vi "MAIN.vi"() -> ()   [LabVIEW 2019]
uses:
  TypeDefs/Estados_flujo_Debug.ctl
  TypeDefs/CLUSTER_CONTROLES_INDICADORES.ctl
  TypeDefs/TAREAS.ctl
  SHARED TYPES/Acciones_UI.ctl
  <vilib>/Utility/error.llb/Error Cluster From Error Code.vi
  <vilib>/ErrorRing/Error Ring.xnode
  SHARED TYPES/SHARED TYPES.lvlib
  SHARED VI'S/SHARED VI'S.lvlib
  MOVIMIENTO_CABEZAL/LABVIEW_MOVIMIENTO_ABSOLUTO/MAIN_call.vi
panel:
  in  "Tab Control":enum32{"Page 1", "Page 2"}(tab)
  in  "TEST ASICS":bool
  in  "LEER QR":bool
  out "LABVIEW MESSAGES":string
  in  "MOVER ASICS":bool
  in  "CALIBRACION":bool
  in  "Exit":bool
  in  "INICIAR COM":bool
  out "DISPOSITIVO CONECTADO":string
  out "ARDUINO MESSAGES":string
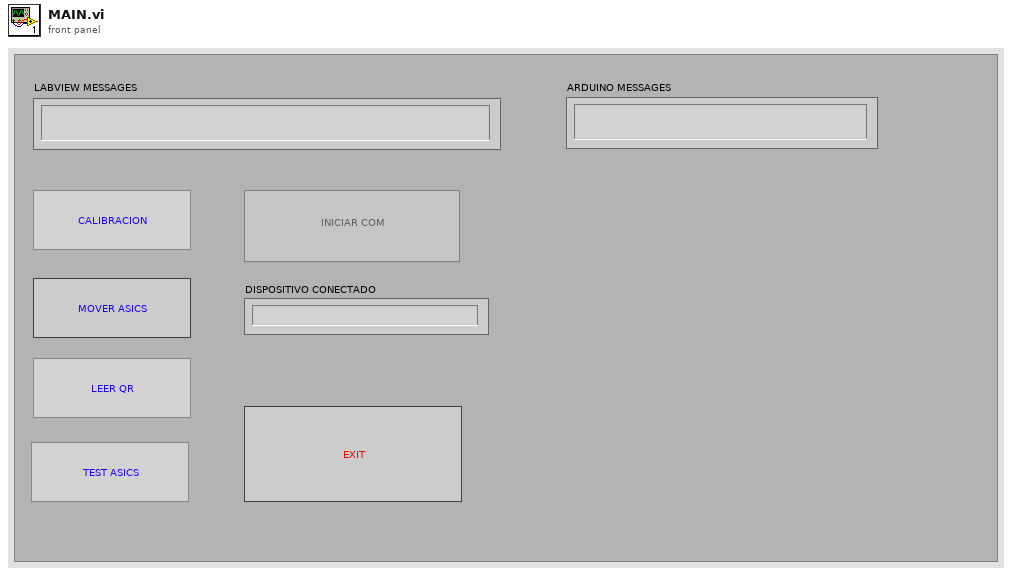
[diagram p1: front panel]
types:
  T1 = typedef "TAREAS.ctl" = enum16{"NINGUNA", "TEST ASICS", "CALIBRACION", "MOVER ASICS", "LEER QR"}
  T2 = typedef "CLUSTER_CONTROLES_INDICADORES.ctl" = cluster{"TEST ASICS":refnum<vi>, "MOVER ASICS":refnum<vi>, "LEER QR'S":refnum<vi>, "MESSAGES":refnum<vi>, "INICIAR COM":refnum<vi>, "stop":refnum<vi>, "CALIBRACION":refnum<vi>}
  T3 = typedef "Estados_flujo_Debug.ctl" = enum16{"Init", "Sesiones Visa abiertas?", "Iniciar Visa Arduino", "Esperar Evento", "Tarea", "Ping to Arduino", "Wait to flag", "Exit", "Error?"}
  T4 = typedef "SHARED TYPES.lvlib/Acciones_UI.ctl" = enum16{"Activar", "Desactivar", "Reiniciar default"}
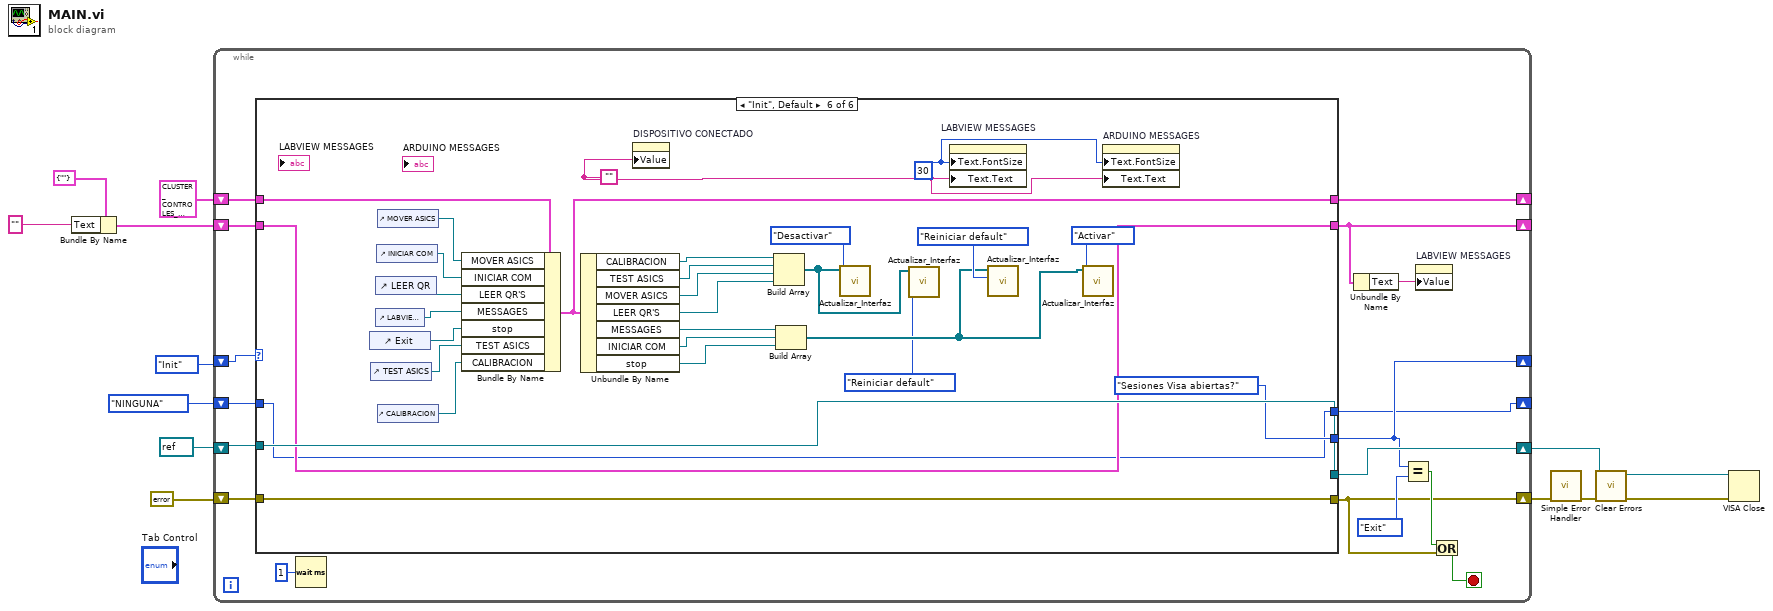
[diagram p0: block diagram]
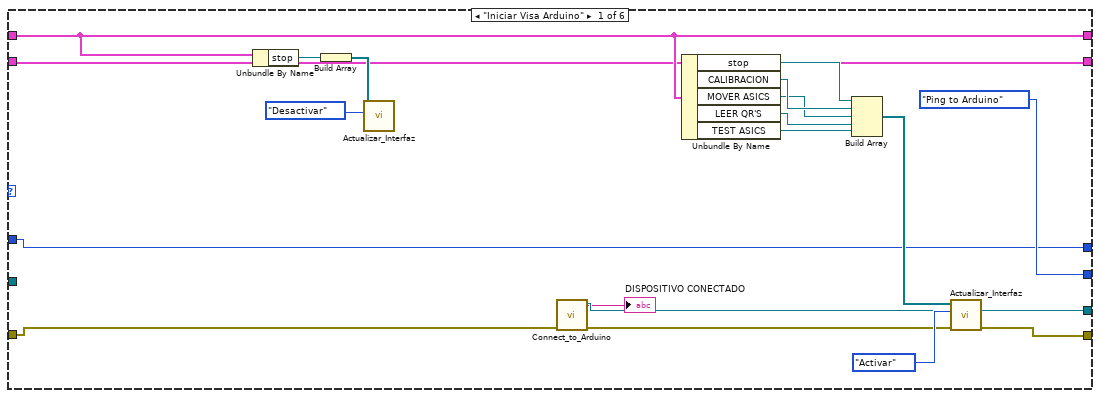
[diagram p2: hidden frame]
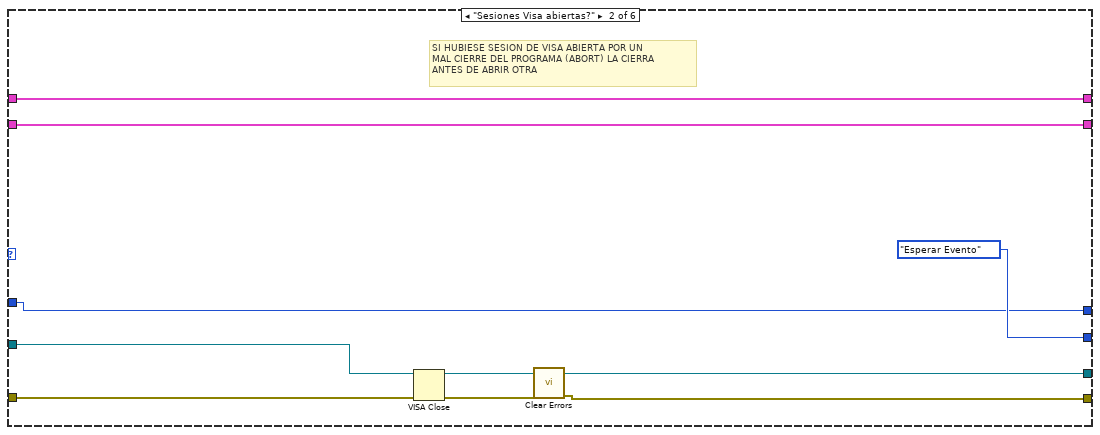
[diagram p3: hidden frame]
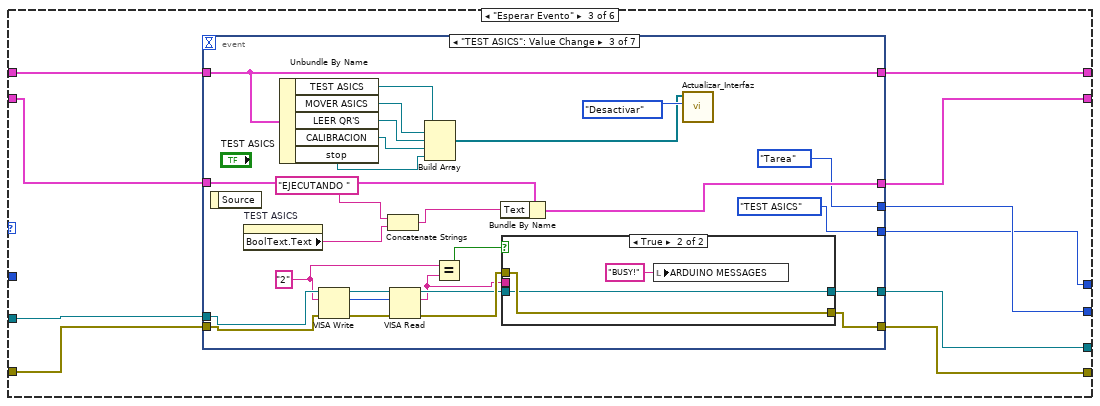
[diagram p4: hidden frame]
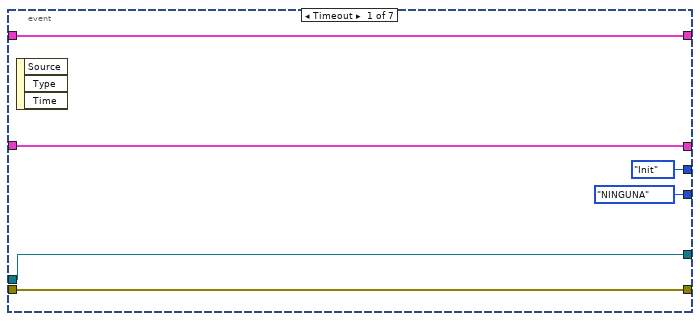
[diagram p5: hidden frame]
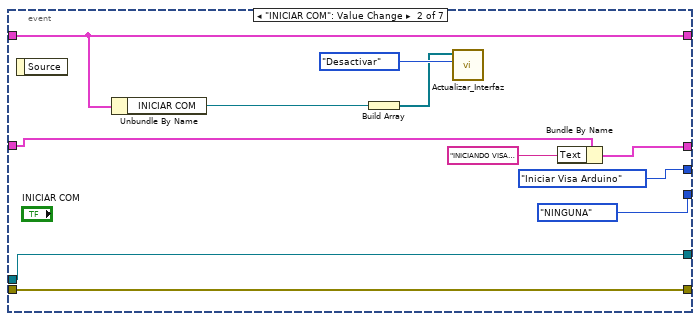
[diagram p6: hidden frame]
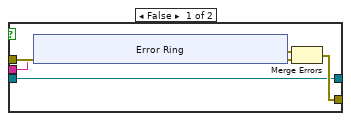
[diagram p7: hidden frame]
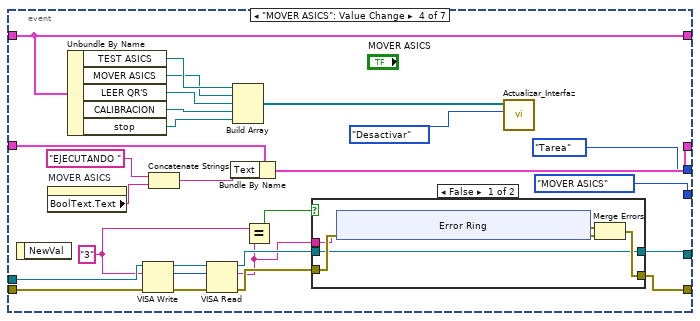
[diagram p8: hidden frame]
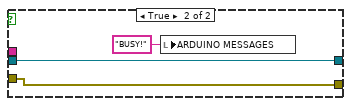
[diagram p9: hidden frame]
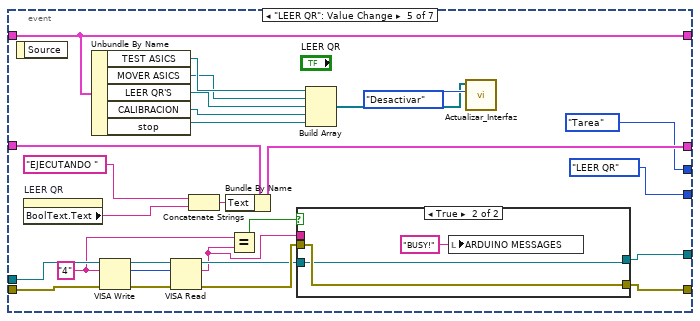
[diagram p10: hidden frame]
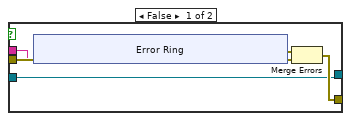
[diagram p11: hidden frame]
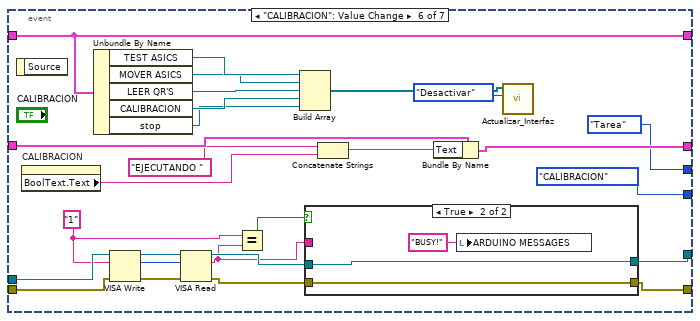
[diagram p12: hidden frame]
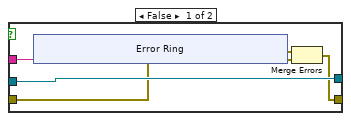
[diagram p13: hidden frame]
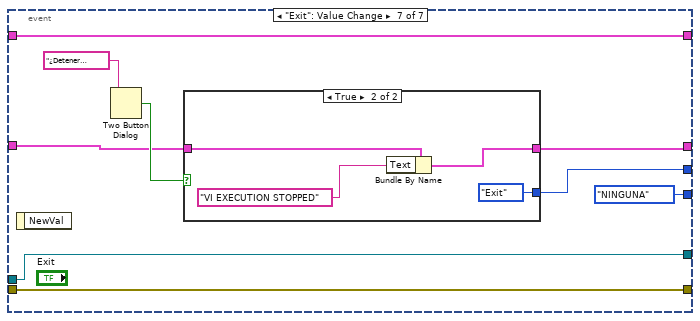
[diagram p14: hidden frame]
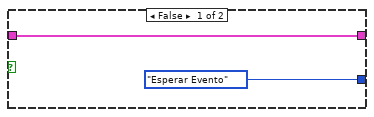
[diagram p15: hidden frame]
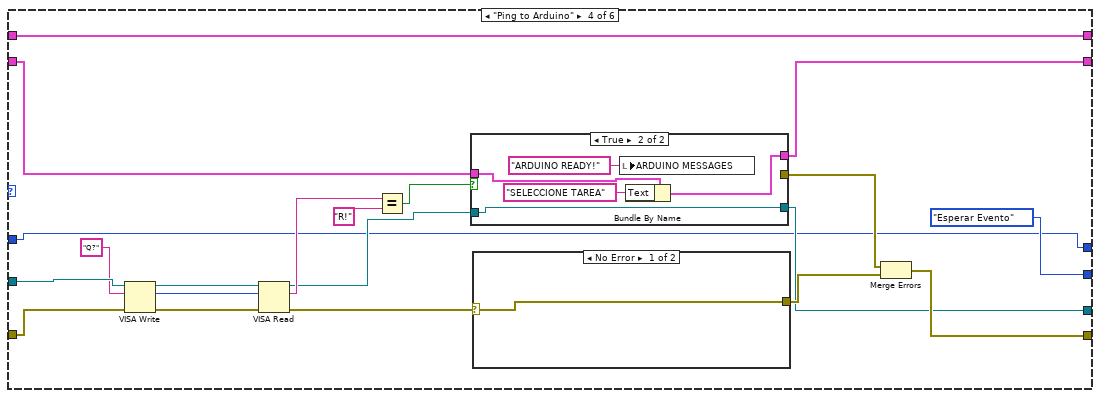
[diagram p16: hidden frame]
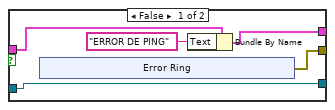
[diagram p17: hidden frame]
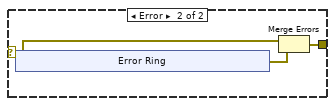
[diagram p18: hidden frame]
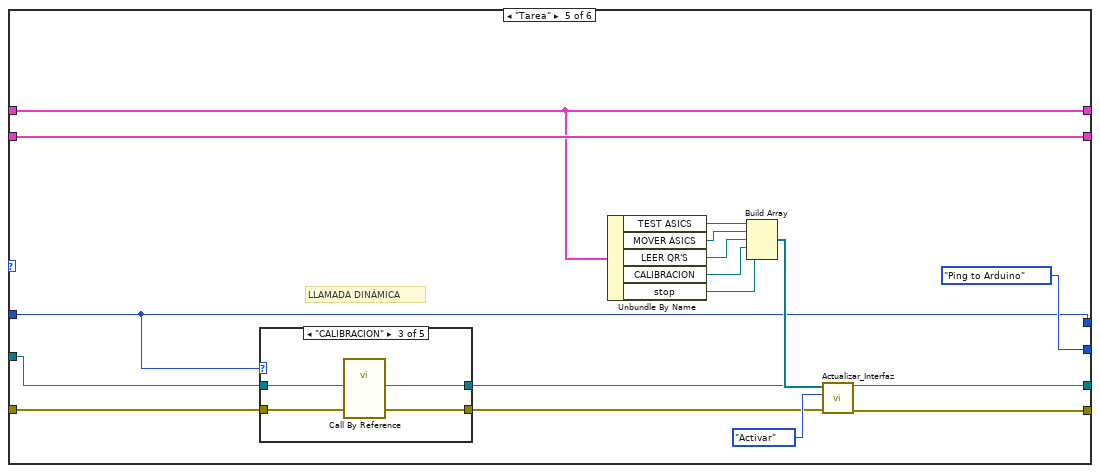
[diagram p19: hidden frame]
diagram:
  n1 = Bundle By Name(cluster=cluster{"Text":string} {"Text"=""}, "Text"="" ("element")) -> (w3:cluster{"Text":string})
  n2 = while {
    shift-right: [w20] -> w7
    shift-left: errorcluster {"status"=FALSE, "code"=0, "source"=""} ("error out") -> [w29]
    shift-right: [w23] -> w11
    shift-left: refnum<visa-resource-name> refnum ("VISA resource name out") -> [w24]
    shift-right: [w25] -> _
    shift-left: T2 {"TEST ASICS"=refnum, "MOVER ASICS"=refnum, "LEER QR'S"=refnum, "MESSAGES"=refnum, "INICIAR COM"=refnum, "stop"=refnum, "CALIBRACION"=refnum} ("INDICADORES_CONTROLES") -> [w26]
    shift-right: [w17] -> _
    shift-left: w3 -> [w19]
    shift-right: [w15] -> _
    shift-left: Estados_flujo_Debug."Init" -> [w16]
    shift-right: [w13] -> _
    shift-left: TAREAS."NINGUNA" ("TAREAS") -> [w14]
    stop <- w28 stop-if-true
    n3 = case shown="\"Init\", Default" w16 {
      tunnel: w29 -> [w33 w56 w65 w283 w325 w337]
      tunnel: [w41 w52 w64 w275 w314 w337] -> w20
      tunnel: [w40 w53 w62 w272 w313 w346] -> w23
      tunnel: w26 -> [w42 w54 w59 w271 w322 w347]
      tunnel: [w42 w54 w66 w271 w322 w345] -> w25
      tunnel: w24 -> [_ w53 w63 w286 w324 w346]
      tunnel: w19 -> [w34 w51 w61 w270 w326 w338]
      tunnel: [w34 w51 w60 w269 w326 w338] -> w17
      tunnel: [Estados_flujo_Debug."Ping to Arduino" Estados_flujo_Debug."Esperar Evento" ("Enum") w58 Estados_flujo_Debug."Esperar Evento" Estados_flujo_Debug."Ping to Arduino" ("Enum") Estados_flujo_Debug."Sesiones Visa abiertas?"] -> w15
      tunnel: w14 -> [w30 w49 _ w267 w311 w333]
      tunnel: [w30 w49 w57 w267 w311 w333] -> w13
      frame "Iniciar Visa Arduino" {
        n4 = Unbundle By Name(w42) -> ("stop"=w48:refnum<vi>)
        n5 = Build Array(w48) -> (w47:refnum<vi>[])
        n6 = call "Actualizar_Interfaz.vi"("Enum"=Acciones_UI."Desactivar", "Controls"=w47) -> ()  [unwired: 9 in, 1 out]
        n7 = call "Connect_to_Arduino.vi"("error in (no error)"=w33) -> ("error out"=w32:errorcluster, "DISPOSITIVO CONECTADO"=→"DISPOSITIVO CONECTADO":string, "VISA Refnum out"=w40:refnum<visa-resource-name>)  [unwired: 8 in]
        n8 = Unbundle By Name(w42) -> ("stop"=w45:refnum<vi>, "CALIBRACION"=w39:refnum<vi>, "MOVER ASICS"=w38:refnum<vi>, "LEER QR'S"=w37:refnum<vi>, "TEST ASICS"=w36:refnum<vi>)
        n9 = Build Array(w45, w39, w38, w37, w36) -> (w44:refnum<vi>[])
        n10 = call "Actualizar_Interfaz.vi"("error in (no error)"=w32, "Enum"=Acciones_UI."Activar", "Controls"=w44) -> ("error out"=w41:errorcluster)  [unwired: 8 in]
      }
      frame "Sesiones Visa abiertas?" {
        # "SI HUBIESE SESION DE VISA ABIERTA POR UN \nMAL CIERRE DEL PROGRAMA (ABORT) LA CIERRA\nANTES DE ABRIR OTRA"
        n11 = VISA Close(VISA resource name=w53, error in (no error)=w56) -> (error out=w55:errorcluster)
        n12 = call <vilib>:"Clear Errors.vi"("error in (no error)"=w55) -> ("error out"=w52:errorcluster)  [unwired: 5 in, 1 out]
      }
      frame "Esperar Evento" {
        n13 = event shown="[2] \"TEST ASICS\": Value Change" {
          selector: _ -> [_ _ _ _ _ _ _]
          dyn-events: _ -> [_ _ _ _ _ _ _]
          timeout: _ -> [_ _ _ _ _ _ _]
          tunnel: w59 -> [w72 w80 w101 w143 w185 w226 w260]
          tunnel: [w72 w80 w101 w143 w185 w226 w260] -> w66
          tunnel: w65 -> [w70 w75 w93 w135 w177 w219 w256]
          tunnel: [w70 w75 w89 w129 w171 w213 w256] -> w64
          tunnel: w63 -> [w71 w79 w100 w142 w184 w227 w257]
          tunnel: [w71 w79 w87 w130 w173 w215 w257] -> w62
          tunnel: w61 -> [w69 w77 w96 w137 w179 w224 w255]
          tunnel: [w69 w76 w94 w136 w178 w220 w254] -> w60
          tunnel: [Estados_flujo_Debug."Init" Estados_flujo_Debug."Iniciar Visa Arduino" Estados_flujo_Debug."Tarea" Estados_flujo_Debug."Tarea" Estados_flujo_Debug."Tarea" Estados_flujo_Debug."Tarea" w253] -> w58
          tunnel: [TAREAS."NINGUNA" ("TAREAS") TAREAS."NINGUNA" ("TAREAS") TAREAS."TEST ASICS" ("TAREAS") TAREAS."MOVER ASICS" ("TAREAS") TAREAS."LEER QR" ("TAREAS") TAREAS."CALIBRACION" ("TAREAS") TAREAS."NINGUNA" ("TAREAS")] -> w57
          event Timeout {
            n14 = event-data() -> ()  [unwired: 1 in, 3 out]
          }
          event "INICIAR COM": Value Change {
            n15 = event-data() -> ()  [unwired: 1 in, 1 out]
            n16 = Unbundle By Name(w80) -> ("INICIAR COM"=w82:refnum<vi>)
            n17 = Build Array(w82) -> (w81:refnum<vi>[])
            n18 = call "Actualizar_Interfaz.vi"("Enum"=Acciones_UI."Desactivar", "Controls"=w81) -> ()  [unwired: 9 in, 1 out]
            n19 = Bundle By Name(cluster=w77, "Text"="INICIANDO VISA Y ARDUINO.....ESPERE" ("String")) -> (w76:cluster{"Text":string})
          }
          event "TEST ASICS": Value Change {
            w91 = "2" ("write buffer")
            n20 = event-data() -> ()  [unwired: 1 in, 1 out]
            n21 = property on="TEST ASICS" class="Bool"() -> ("BoolText.Text"=w98:string)  [unwired: 2 in, 2 out]
            n22 = Unbundle By Name(w101) -> ("TEST ASICS"=w107:refnum<vi>, "MOVER ASICS"=w106:refnum<vi>, "LEER QR'S"=w105:refnum<vi>, "CALIBRACION"=w104:refnum<vi>, "stop"=w99:refnum<vi>)
            n23 = VISA Write(VISA resource name=w100, write buffer=w91, error in (no error)=w93) -> (VISA resource name out=w109:refnum<visa-resource-name>, return count=w108:u32, error out=w110:errorcluster)
            n24 = Concatenate Strings("EJECUTANDO " ("string"), w98) -> (w97:string)
            n25 = VISA Read(VISA resource name=w109, byte count=w108, error in (no error)=w110) -> (VISA resource name out=w88:refnum<visa-resource-name>, read buffer=w86:string, error out=w90:errorcluster)  [unwired: 1 out]
            n26 = Build Array(w107, w106, w105, w104, w99) -> (w102:refnum<vi>[])
            n27 = Equal?(x=w91, y=w86) -> (x = y?=w92:bool)
            n28 = Bundle By Name(cluster=w96, "Text"=w97) -> (w94:cluster{"Text":string})
            n29 = case shown="True" w92 {
              tunnel: [w115 w124] -> w89
              tunnel: w90 -> [w113 w124]
              tunnel: w88 -> [w112 w123]
              tunnel: [w112 w123] -> w87
              tunnel: w86 -> [w111 _]
              frame False {
                n30 = xnode "Error Ring"("parameter 0"=w111) -> ("error out"=w114:errorcluster)
                n31 = Merge Errors(w114, w113) -> (w115:errorcluster)
              }
              frame True {
                n32 = local write "ARDUINO MESSAGES"("BUSY!" ("ARDUINO MESSAGES")) -> ()
              }
            }
            n33 = call "Actualizar_Interfaz.vi"("Enum"=Acciones_UI."Desactivar", "Controls"=w102) -> ()  [unwired: 9 in, 1 out]
          }
          event "MOVER ASICS": Value Change {
            w132 = "3" ("write buffer")
            n34 = event-data() -> ()  [unwired: 1 in, 1 out]
            n35 = property on="MOVER ASICS" class="Bool"() -> ("BoolText.Text"=w140:string)  [unwired: 2 in, 2 out]
            n36 = Unbundle By Name(w143) -> ("TEST ASICS"=w149:refnum<vi>, "MOVER ASICS"=w148:refnum<vi>, "LEER QR'S"=w147:refnum<vi>, "CALIBRACION"=w146:refnum<vi>, "stop"=w141:refnum<vi>)
            n37 = VISA Write(VISA resource name=w142, write buffer=w132, error in (no error)=w135) -> (VISA resource name out=w151:refnum<visa-resource-name>, return count=w150:u32, error out=w152:errorcluster)
            n38 = Concatenate Strings("EJECUTANDO " ("string"), w140) -> (w138:string)
            n39 = VISA Read(VISA resource name=w151, byte count=w150, error in (no error)=w152) -> (VISA resource name out=w131:refnum<visa-resource-name>, read buffer=w128:string, error out=w133:errorcluster)  [unwired: 1 out]
            n40 = Bundle By Name(cluster=w137, "Text"=w138) -> (w136:cluster{"Text":string})
            n41 = Build Array(w149, w148, w147, w146, w141) -> (w144:refnum<vi>[])
            n42 = Equal?(x=w132, y=w128) -> (x = y?=w134:bool)
            n43 = case shown="False" w134 {
              tunnel: [w157 w167] -> w129
              tunnel: w133 -> [w155 w167]
              tunnel: [w154 w165] -> w130
              tunnel: w131 -> [w154 w165]
              tunnel: w128 -> [w153 _]
              frame False {
                n44 = xnode "Error Ring"("parameter 0"=w153) -> ("error out"=w156:errorcluster)
                n45 = Merge Errors(w156, w155) -> (w157:errorcluster)
              }
              frame True {
                n46 = local write "ARDUINO MESSAGES"("BUSY!" ("ARDUINO MESSAGES")) -> ()
              }
            }
            n47 = call "Actualizar_Interfaz.vi"("Enum"=Acciones_UI."Desactivar", "Controls"=w144) -> ()  [unwired: 9 in, 1 out]
          }
          event "LEER QR": Value Change {
            w172 = "4" ("write buffer")
            n48 = event-data() -> ()  [unwired: 1 in, 1 out]
            n49 = property on="LEER QR" class="Bool"() -> ("BoolText.Text"=w182:string)  [unwired: 2 in, 2 out]
            n50 = Unbundle By Name(w185) -> ("TEST ASICS"=w191:refnum<vi>, "MOVER ASICS"=w190:refnum<vi>, "LEER QR'S"=w189:refnum<vi>, "CALIBRACION"=w188:refnum<vi>, "stop"=w183:refnum<vi>)
            n51 = VISA Write(VISA resource name=w184, write buffer=w172, error in (no error)=w177) -> (VISA resource name out=w193:refnum<visa-resource-name>, return count=w192:u32, error out=w194:errorcluster)
            n52 = VISA Read(VISA resource name=w193, byte count=w192, error in (no error)=w194) -> (VISA resource name out=w174:refnum<visa-resource-name>, read buffer=w170:string, error out=w175:errorcluster)  [unwired: 1 out]
            n53 = Concatenate Strings("EJECUTANDO " ("string"), w182) -> (w180:string)
            n54 = Bundle By Name(cluster=w179, "Text"=w180) -> (w178:cluster{"Text":string})
            n55 = Equal?(x=w172, y=w170) -> (x = y?=w176:bool)
            n56 = case shown="True" w176 {
              tunnel: [w199 w209] -> w171
              tunnel: w175 -> [w197 w209]
              tunnel: [w196 w207] -> w173
              tunnel: w174 -> [w196 w207]
              tunnel: w170 -> [w195 _]
              frame False {
                n57 = xnode "Error Ring"("parameter 0"=w195) -> ("error out"=w198:errorcluster)
                n58 = Merge Errors(w198, w197) -> (w199:errorcluster)
              }
              frame True {
                n59 = local write "ARDUINO MESSAGES"("BUSY!" ("ARDUINO MESSAGES")) -> ()
              }
            }
            n60 = Build Array(w191, w190, w189, w188, w183) -> (w186:refnum<vi>[])
            n61 = call "Actualizar_Interfaz.vi"("Enum"=Acciones_UI."Desactivar", "Controls"=w186) -> ()  [unwired: 9 in, 1 out]
          }
          event "CALIBRACION": Value Change {
            w218 = "1" ("write buffer")
            n62 = event-data() -> ()  [unwired: 1 in, 1 out]
            n63 = property on="CALIBRACION" class="Bool"() -> ("BoolText.Text"=w222:string)  [unwired: 2 in, 2 out]
            n64 = Unbundle By Name(w226) -> ("TEST ASICS"=w233:refnum<vi>, "MOVER ASICS"=w232:refnum<vi>, "LEER QR'S"=w231:refnum<vi>, "CALIBRACION"=w230:refnum<vi>, "stop"=w225:refnum<vi>)
            n65 = VISA Write(VISA resource name=w227, write buffer=w218, error in (no error)=w219) -> (VISA resource name out=w235:refnum<visa-resource-name>, return count=w234:u32, error out=w236:errorcluster)
            n66 = VISA Read(VISA resource name=w235, byte count=w234, error in (no error)=w236) -> (VISA resource name out=w216:refnum<visa-resource-name>, read buffer=w212:string, error out=w214:errorcluster)  [unwired: 1 out]
            n67 = Equal?(x=w218, y=w212) -> (x = y?=w217:bool)
            n68 = Build Array(w233, w232, w231, w230, w225) -> (w228:refnum<vi>[])
            n69 = case shown="True" w217 {
              tunnel: w216 -> [w241 w250]
              tunnel: [w241 w250] -> w215
              tunnel: w214 -> [w240 w249]
              tunnel: [w239 w249] -> w213
              tunnel: w212 -> [w237 _]
              frame False {
                n70 = xnode "Error Ring"("parameter 0"=w237) -> ("error out"=w238:errorcluster)
                n71 = Merge Errors(w238, w240) -> (w239:errorcluster)
              }
              frame True {
                n72 = local write "ARDUINO MESSAGES"("BUSY!" ("ARDUINO MESSAGES")) -> ()
              }
            }
            n73 = Concatenate Strings("EJECUTANDO " ("element"), w222) -> (w221:string)
            n74 = Bundle By Name(cluster=w224, "Text"=w221) -> (w220:cluster{"Text":string})
            n75 = call "Actualizar_Interfaz.vi"("Enum"=Acciones_UI."Desactivar", "Controls"=w228) -> ()  [unwired: 9 in, 1 out]
          }
          event "Exit": Value Change {
            n76 = event-data() -> ()  [unwired: 1 in, 1 out]
            n77 = Two Button Dialog(message="¿Detener ejecución?") -> (T button?=w259:bool)  [unwired: 2 in]
            n78 = case shown="True" w259 {
              tunnel: [Estados_flujo_Debug."Esperar Evento" Estados_flujo_Debug."Exit"] -> w253
              tunnel: w255 -> [w261 w264]
              tunnel: [w261 w263] -> w254
              frame False {
              }
              frame True {
                n79 = Bundle By Name(cluster=w264, "Text"="VI EXECUTION STOPPED" ("MESSAGES")) -> (w263:cluster{"Text":string})
              }
            }
          }
        }
      }
      frame "Ping to Arduino" {
        n80 = VISA Write(VISA resource name=w286, write buffer="Q?", error in (no error)=w283) -> (VISA resource name out=w284:refnum<visa-resource-name>, return count=w282:u32, error out=w281:errorcluster)
        n81 = VISA Read(VISA resource name=w284, byte count=w282, error in (no error)=w281) -> (VISA resource name out=w273:refnum<visa-resource-name>, read buffer=w280:string, error out=w278:errorcluster)  [unwired: 1 out]
        n82 = Equal?(x=w280, y="R!") -> (x = y?=w277:bool)
        n83 = case shown="True" w277 {
          tunnel: [w291 _] -> w274
          tunnel: w273 -> [w290 w300]
          tunnel: [w290 w300] -> w272
          tunnel: w270 -> [w289 w299]
          tunnel: [w287 w298] -> w269
          frame False {
            n84 = xnode "Error Ring"() -> ("error out"=w291:errorcluster)
            n85 = Bundle By Name(cluster=w289, "Text"="ERROR DE PING") -> (w287:cluster{"Text":string})
          }
          frame True {
            n86 = local write "ARDUINO MESSAGES"("ARDUINO READY!" ("ARDUINO MESSAGES")) -> ()
            n87 = Bundle By Name(cluster=w299, "Text"="SELECCIONE TAREA") -> (w298:cluster{"Text":string})
          }
        }
        n88 = case shown="No Error" w278 {
          selector: w278 -> [w302 w304]
          tunnel: [w302 w303] -> w276
          frame No Error {
          }
          frame Error {
            n89 = xnode "Error Ring"() -> ("error out"=w305:errorcluster)
            n90 = Merge Errors(w304, w305) -> (w303:errorcluster)
          }
        }
        n91 = Merge Errors(w274, w276) -> (w275:errorcluster)
      }
      frame "Tarea" {
        # "LLAMADA DINÁMICA"
        n92 = case shown="\"CALIBRACION\"" w311 {
          tunnel: w325 -> [w327 _ w332 _ _]
          tunnel: w324 -> [w328 _ w331 _ _]
          tunnel: [w327 _ w330 _ _] -> w315
          tunnel: [w328 _ w329 _ _] -> w313
          frame "NINGUNA", Default {
          }
          frame "TEST ASICS" {
          }
          frame "CALIBRACION" {
            n93 = call-by-ref "?"("error in (no error)"=w332, "VISA resource name"=w331) -> ("error out"=w330:errorcluster, "VISA resource name 2"=w329:refnum<visa-resource-name>)  [unwired: 10 in, 2 out]
          }
          frame "MOVER ASICS" {
          }
          frame "LEER QR" {
          }
        }
        n94 = Unbundle By Name(w322) -> ("TEST ASICS"=w323:refnum<vi>, "MOVER ASICS"=w321:refnum<vi>, "LEER QR'S"=w320:refnum<vi>, "CALIBRACION"=w319:refnum<vi>, "stop"=w318:refnum<vi>)
        n95 = Build Array(w323, w321, w320, w319, w318) -> (w317:refnum<vi>[])
        n96 = call "Actualizar_Interfaz.vi"("error in (no error)"=w315, "Enum"=Acciones_UI."Activar", "Controls"=w317) -> ("error out"=w314:errorcluster)  [unwired: 8 in]
      }
      frame "Init", Default {
        w336 = ""
        w335 = u32 30 ("Text.Font:Size")
        n97 = control-ref of="Exit"() -> (w360:refnum<vi>)
        n98 = control-ref of="TEST ASICS"() -> (w339:refnum<vi>)
        n99 = control-ref of="LEER QR"() -> (w340:refnum<vi>)
        n100 = control-ref of="LABVIEW MESSAGES"() -> (w359:refnum<vi>)
        n101 = control-ref of="INICIAR COM"() -> (w358:refnum<vi>)
        n102 = control-ref of="MOVER ASICS"() -> (w357:refnum<vi>)
        n103 = control-ref of="CALIBRACION"() -> (w361:refnum<vi>)
        n104 = Bundle By Name(cluster=w347, "MOVER ASICS"=w357, "INICIAR COM"=w358, "LEER QR'S"=w340, "MESSAGES"=w359, "stop"=w360, "TEST ASICS"=w339, "CALIBRACION"=w361) -> (w345:T2)
        n105 = Unbundle By Name(w345) -> ("CALIBRACION"=w354:refnum<vi>, "TEST ASICS"=w353:refnum<vi>, "MOVER ASICS"=w352:refnum<vi>, "LEER QR'S"=w351:refnum<vi>, "MESSAGES"=w350:refnum<vi>, "INICIAR COM"=w349:refnum<vi>, "stop"=w348:refnum<vi>)
        n106 = property on="DISPOSITIVO CONECTADO" class="Str"("Value"=w336) -> ()  [unwired: 2 in, 2 out]
        n107 = Build Array(w354, w353, w352, w351) -> (w341:refnum<vi>[])
        n108 = Build Array(w350, w349, w348) -> (w344:refnum<vi>[])
        n109 = call "Actualizar_Interfaz.vi"("Enum"=Acciones_UI."Desactivar", "Controls"=w341) -> ()  [unwired: 9 in, 1 out]
        n110 = call "Actualizar_Interfaz.vi"("Enum"=Acciones_UI."Reiniciar default", "Controls"=w341) -> ()  [unwired: 9 in, 1 out]
        n111 = property on="LABVIEW MESSAGES" class="Str"("Text.FontSize"=w335, "Text.Text"=w336) -> ()  [unwired: 2 in, 2 out]
        n112 = call "Actualizar_Interfaz.vi"("Enum"=Acciones_UI."Reiniciar default", "Controls"=w344) -> ()  [unwired: 9 in, 1 out]
        n113 = call "Actualizar_Interfaz.vi"("Enum"=Acciones_UI."Activar", "Controls"=w344) -> ()  [unwired: 9 in, 1 out]
        n114 = property on="ARDUINO MESSAGES" class="Str"("Text.FontSize"=w335, "Text.Text"=w336) -> ()  [unwired: 2 in, 2 out]
      }
    }
    n115 = Wait (ms)(milliseconds to wait=u32 1) -> ()  [unwired: 1 out]
    n116 = Unbundle By Name(w17) -> ("Text"=w18:string)
    n117 = Equal?(x=w15, y=Estados_flujo_Debug."Exit") -> (x = y?=w21:bool)
    n118 = property on="LABVIEW MESSAGES" class="Str"("Value"=w18) -> ()  [unwired: 2 in, 2 out]
    n119 = Or(x=w21, y=w20) -> (x .or. y?=w28:bool)
  }
  n120 = call <vilib>:"Simple Error Handler.vi"("error in (no error)"=w7) -> ("error out"=w6:errorcluster)  [unwired: 4 in, 4 out]
  n121 = call <vilib>:"Clear Errors.vi"("error in (no error)"=w6) -> ("error out"=w10:errorcluster)  [unwired: 5 in, 1 out]
  n122 = VISA Close(VISA resource name=w11, error in (no error)=w10) -> ()  [unwired: 1 out]
